vi "Temp 3-6.vi"() -> ()   [LabVIEW 2014]
uses:
  Control 1.ctl
panel:
  out "?":dbl(slide) scale=0.0..100.0
  in  "?":dbl(slide) scale=0.0..50.0
  in  "?":T1(ring)
  in  "On/Off":T2
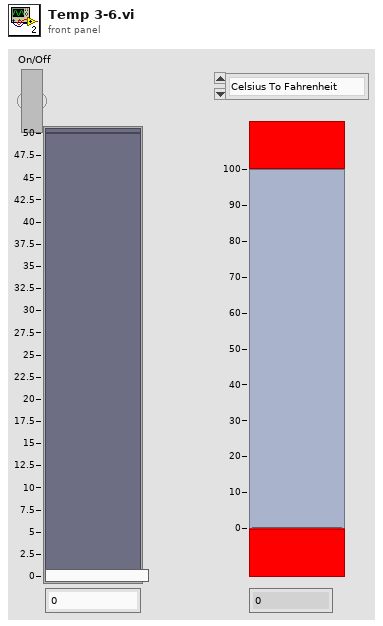
[diagram p1: front panel]
types:
  T1 = enum16{"Celsius To Fahrenheit", "Fahrenheit To Celsius", "Celsius To Kelvin", "Fahrenheit to Kelvin"}
  T2 = typedef "Control 1.ctl" = bool
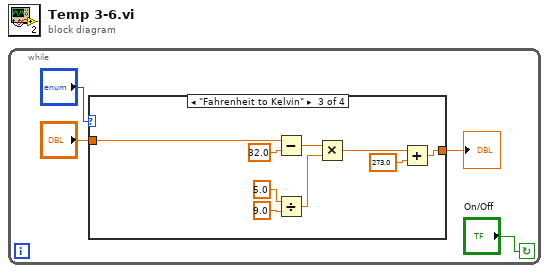
[diagram p0: block diagram]
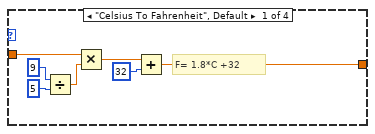
[diagram p2: hidden frame]
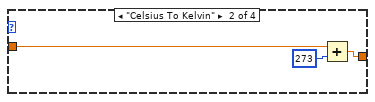
[diagram p3: hidden frame]
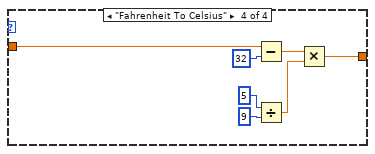
[diagram p4: hidden frame]
diagram:
  n1 = while {
    stop <- "On/Off" continue-if-true
    n2 = case shown="\"Fahrenheit to Kelvin\"" "?" {
      tunnel: "?" -> [w11 w13 w22 w27]
      tunnel: [w5 w12 w15 w24] -> w1
      frame "Celsius To Fahrenheit", Default {
        # "F= 1.8*C +32"
        n3 = Divide(x=9, y=5) -> (x/y=w10:dbl)
        n4 = Multiply(x=w11, y=w10) -> (x*y=w7:dbl)
        n5 = Add(x=w7, y=32) -> (x+y=w5:dbl)
      }
      frame "Celsius To Kelvin" {
        n6 = Add(x=w13, y=273) -> (x+y=w12:dbl)
      }
      frame "Fahrenheit to Kelvin" {
        n7 = Subtract(x=w22, y=32.0) -> (x-y=w21:dbl)
        n8 = Divide(x=5.0, y=9.0) -> (x/y=w20:dbl)
        n9 = Multiply(x=w21, y=w20) -> (x*y=w17:dbl)
        n10 = Add(x=w17, y=273.0) -> (x+y=w15:dbl)
      }
      frame "Fahrenheit To Celsius" {
        n11 = Subtract(x=w27, y=32) -> (x-y=w25:dbl)
        n12 = Divide(x=5, y=9) -> (x/y=w30:dbl)
        n13 = Multiply(x=w25, y=w30) -> (x*y=w24:dbl)
      }
    }
    "?" <- w1
  }
